vi "Virtual Voltmeter test.vi"() -> ()   [LabVIEW 2023]
uses:
  Voltmeter/Virtual Voltmeter/Virtual Voltmeter.lvclass
  Devices/PXIe-5172/Configurations/Voltmeter CFG/Voltmeter CFG/Voltmeter CFG.lvclass
  D:/git/HAL/Interfaces/IConfigure/IConfigure.lvclass
  Devices/PXIe-5172/PXIe-5172.lvclass
  Voltmeter/Virtual Voltmeter/Virtual Voltmeter.lvclass/Virtual Voltmeter.ctl
  Devices/PXIe-5172/PXIe-5172Ref/PXIe-5172Ref.lvclass
  D:/git/HAL/Interfaces/IRead Voltage Multichannel/IRead Voltage from Channel.lvclass
  <userlib>/_OpenG.lib/file/file.llb/openg_file.lvlib
panel:
  out "Waveform Chart 2":dbl(graph)
  out "filenames":string[](array[string])
  out "error out":errorcluster
  out "Waveform Chart":dbl(graph)
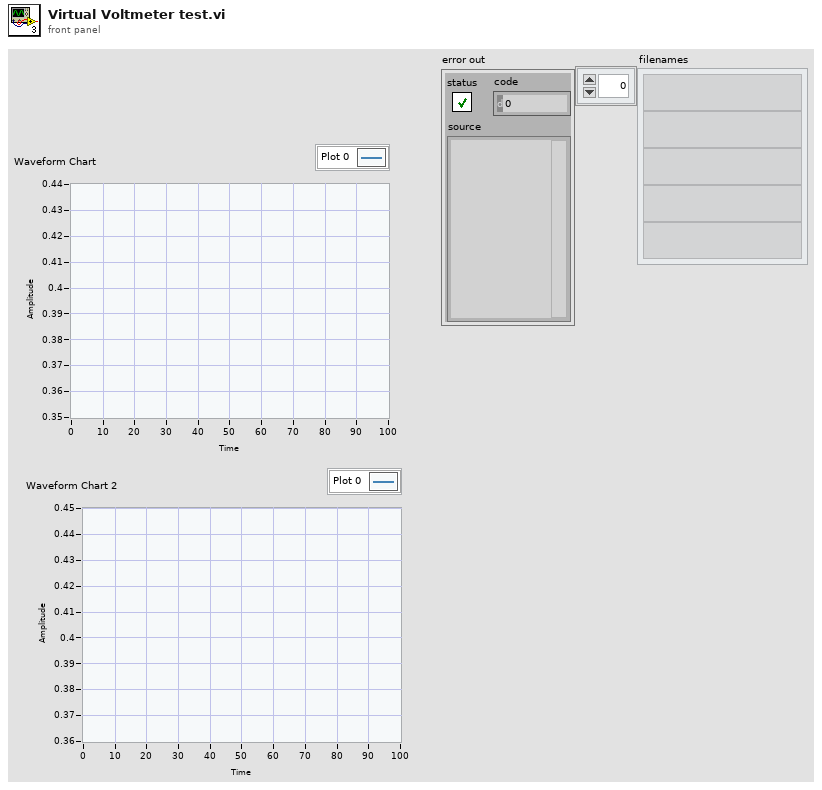
[diagram p1: front panel]
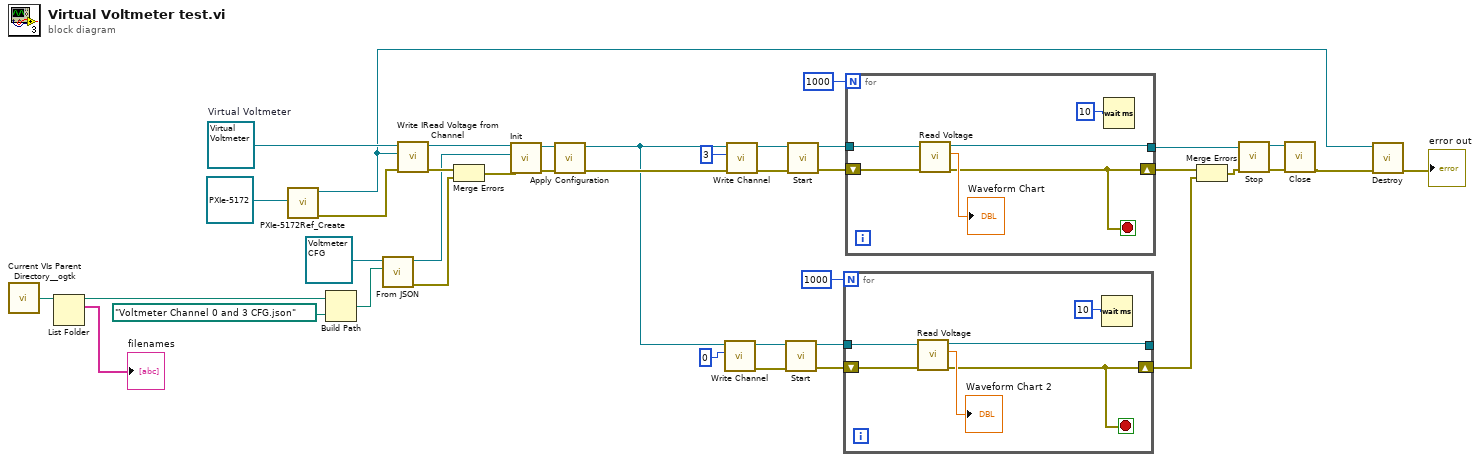
[diagram p0: block diagram]
diagram:
  w39 = refnum<class "Virtual Voltmeter.lvclass"> refnum  # Virtual Voltmeter
  n1 = call <userlib>:"Current VIs Parent Directory__ogtk.vi"() -> ("Parent Directory (+ Relative)"=w21:path)  [unwired: 5 in]
  n2 = List Folder(path=w21) -> (path out=w20:path, filenames=→"filenames":string[])  [unwired: 3 in, 2 out]
  n3 = call "PXIe-5172Ref_Create.vi"("PXIe-5172.lvclass"=refnum<class "PXIe-5172.lvclass"> refnum ("PXIe-5172.lvlib:PXIe-5172.lvclass")) -> ("Error Out"=w32:errorcluster, "reference out"=w7:refnum<class "PXIe-5172Ref.lvclass">)  [unwired: 9 in]
  n4 = Build Path(base path=w20, name or relative path=path "Voltmeter Channel 0 and 3 CFG.json") -> (appended path=w18:path)
  n5 = call-dynamic "From JSON.vi"("JSON Config"=w18, "object in"=refnum<class "Voltmeter CFG.lvclass"> refnum ("PXIe-5172.lvlib:Voltmeter CFG.lvclass")) -> ("error out"=w4:errorcluster, "object out"=w8:refnum<class "Voltmeter CFG.lvclass">)  [unwired: 8 in]
  n6 = call "Write IRead Voltage from Channel.vi"("error in (no error)"=w32, "IRead Voltage from Channel"=w7, "Virtual Voltmeter in"=w39) -> ("error out"=w34:errorcluster, "Virtual Voltmeter out"=w35:refnum<class "Virtual Voltmeter.lvclass">)  [unwired: 7 in]
  n7 = Merge Errors(w34, w4) -> (w5:errorcluster)
  n8 = call-dynamic "Init.vi"("error in"=w5, "IConfigure"=w8, "Virtual Voltmeter in"=w35) -> ("error out"=w38:errorcluster, "Virtual Voltmeter out"=w16:refnum<class "Virtual Voltmeter.lvclass">)  [unwired: 7 in]
  n9 = call-dynamic "Apply Configuration.vi"("error in (no error)"=w38, "Virtual Voltmeter in"=w16) -> ("error out"=w17:errorcluster, "Virtual Voltmeter out"=w6:refnum<class "Virtual Voltmeter.lvclass">)  [unwired: 8 in]
  n10 = call "Write Channel.vi"("Channel"=u8 0, "Virtual Voltmeter in"=w6) -> ("error out"=w10:errorcluster, "Virtual Voltmeter out"=w11:refnum<class "Virtual Voltmeter.lvclass">)  [unwired: 8 in]
  n11 = call "Write Channel.vi"("error in (no error)"=w17, "Channel"=u8 3, "Virtual Voltmeter in"=w6) -> ("error out"=w31:errorcluster, "Virtual Voltmeter out"=w30:refnum<class "Virtual Voltmeter.lvclass">)  [unwired: 7 in]
  n12 = call-dynamic "Start.vi"("error in"=w10, "Virtual Voltmeter in"=w11) -> ("error out"=w14:errorcluster, "Virtual Voltmeter out"=w13:refnum<class "Virtual Voltmeter.lvclass">)  [unwired: 8 in]
  n13 = call-dynamic "Start.vi"("error in"=w31, "Virtual Voltmeter in"=w30) -> ("error out"=w27:errorcluster, "Virtual Voltmeter out"=w28:refnum<class "Virtual Voltmeter.lvclass">)  [unwired: 8 in]
  n14 = for {
    N: 1000 -> [_]
    tunnel: w13 -> [w44]
    tunnel: [w41] -> _
    shift-right: [w40] -> w2
    shift-left: w14 -> [w43]
    stop <- w40 stop-if-true
    n15 = call-dynamic "Read Voltage.vi"("error in (no error)"=w43, "Virtual Voltmeter in"=w44) -> ("error out"=w40:errorcluster, "Voltage"=→"Waveform Chart 2":dbl, "Virtual Voltmeter out"=w41:refnum<class "Virtual Voltmeter.lvclass">)  [unwired: 7 in]
    n16 = Wait (ms)(milliseconds to wait=u32 10) -> ()  [unwired: 1 out]
  }
  n17 = for {
    N: 1000 -> [_]
    tunnel: w28 -> [w50]
    tunnel: [w47] -> w25
    shift-right: [w46] -> w26
    shift-left: w27 -> [w49]
    stop <- w46 stop-if-true
    n18 = call-dynamic "Read Voltage.vi"("error in (no error)"=w49, "Virtual Voltmeter in"=w50) -> ("error out"=w46:errorcluster, "Voltage"=→"Waveform Chart":dbl, "Virtual Voltmeter out"=w47:refnum<class "Virtual Voltmeter.lvclass">)  [unwired: 7 in]
    n19 = Wait (ms)(milliseconds to wait=u32 10) -> ()  [unwired: 1 out]
  }
  n20 = Merge Errors(w26, w2) -> (w3:errorcluster)
  n21 = call-dynamic "Stop.vi"("error in"=w3, "Virtual Voltmeter in"=w25) -> ("error out"=w23:errorcluster, "Virtual Voltmeter out"=w24:refnum<class "Virtual Voltmeter.lvclass">)  [unwired: 8 in]
  n22 = call-dynamic "Close.vi"("error in (no error)"=w23, "Virtual Voltmeter in"=w24) -> ("error out"=w1:errorcluster)  [unwired: 8 in, 1 out]
  n23 = call-dynamic "Destroy.vi"("Error In"=w1, "reference in"=w7) -> ("Error Out"=→"error out":errorcluster)  [unwired: 8 in, 1 out]
